vi "Ctor.vi"(8 "error in (no error)":errorcluster, 11 "Ready Notifier":refnum<notifier>) -> (0 "error out":errorcluster, 3 "App out":refnum<class "App.lvclass">)   [LabVIEW 2020, in "PicoG-App.lvlib" / "App.lvclass"]
uses:
  App.lvclass
  App.lvclass/App.ctl
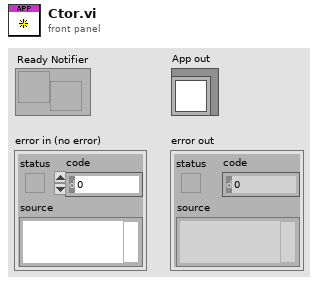
[diagram p1: front panel]
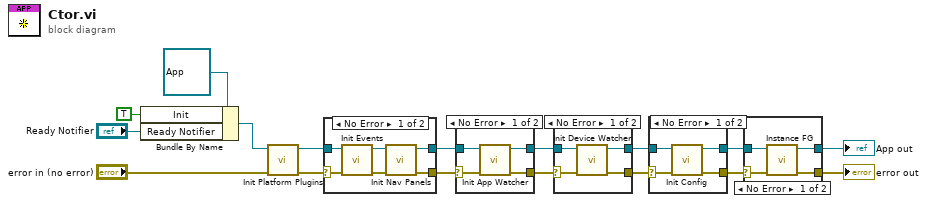
[diagram p0: block diagram]
diagram:
  n1 = Bundle By Name(cluster=refnum<class "App.lvclass"> refnum ("App in"), "Init"=TRUE, "Ready Notifier"="Ready Notifier") -> (w13:refnum<class "App.lvclass">)
  n2 = call "Init Platform Plugins.vi"("error in (no error)"="error in (no error)", "App in"=w13) -> ("error out"=w2:errorcluster, "App out"=w1:refnum<class "App.lvclass">)  [unwired: 8 in]
  n3 = case shown="No Error" w2 {
    selector: w2 -> [w21 w25]
    tunnel: w1 -> [w20 w24]
    tunnel: [w19 w24] -> w12
    tunnel: [w18 w25] -> w11
    frame No Error {
      n4 = call "Init Events.vi"("error in (no error)"=w21, "App in"=w20) -> ("error out"=w22:errorcluster, "App out"=w23:refnum<class "App.lvclass">)  [unwired: 8 in]
      n5 = call "Init Nav Panels.vi"("error in (no error)"=w22, "App in"=w23) -> ("error out"=w18:errorcluster, "App out"=w19:refnum<class "App.lvclass">)  [unwired: 8 in]
    }
    frame Error {
    }
  }
  n6 = case shown="No Error" w11 {
    selector: w11 -> [w28 w30]
    tunnel: [w27 w30] -> w9
    tunnel: [w26 w31] -> w10
    tunnel: w12 -> [w29 w31]
    frame No Error {
      n7 = call "Init App Watcher.vi"("error in (no error)"=w28, "App in"=w29) -> ("error out"=w27:errorcluster, "App out"=w26:refnum<class "App.lvclass">)  [unwired: 8 in]
    }
    frame Error {
    }
  }
  n8 = case shown="No Error" w9 {
    selector: w9 -> [w35 w36]
    tunnel: [w32 w36] -> w6
    tunnel: [w33 w37] -> w5
    tunnel: w10 -> [w34 w37]
    frame No Error {
      n9 = call "Init Device Watcher.vi"("error in (no error)"=w35, "App in"=w34) -> ("error out"=w32:errorcluster, "App out"=w33:refnum<class "App.lvclass">)  [unwired: 8 in]
    }
    frame Error {
    }
  }
  n10 = case shown="No Error" w6 {
    selector: w6 -> [w39 w42]
    tunnel: [w41 w42] -> w3
    tunnel: [w40 w43] -> w4
    tunnel: w5 -> [w38 w43]
    frame No Error {
      n11 = call "Init Config.vi"("error in (no error)"=w39, "App in"=w38) -> ("error out"=w41:errorcluster, "App out"=w40:refnum<class "App.lvclass">)  [unwired: 8 in]
    }
    frame Error {
    }
  }
  n12 = case shown="No Error" w3 {
    selector: w3 -> [w46 w48]
    tunnel: [w44 w48] -> w8
    tunnel: [w45 w49] -> w7
    tunnel: w4 -> [w47 w49]
    frame No Error {
      n13 = call "Instance FG.vi"("error in (no error)"=w46, "App in"=w47) -> ("error out"=w44:errorcluster, "App out"=w45:refnum<class "App.lvclass">)  [unwired: 8 in]
    }
    frame Error {
    }
  }
  "error out" <- w8
  "App out" <- w7
